vi "LVCAM Msg Drop.vi"(10 "Remaining Elements":refnum<class "Msg.lvclass">[](array[class]), 11 "Self Actor in":refnum<class "Self Actor.lvclass">) -> ()   [LabVIEW 2021, in "LVCAM.lvlib" / "Self Actor.lvclass"]
uses:
  Self Actor.lvclass
  Msg/Msg.lvclass
  Self Actor.lvclass/Self Actor.ctl
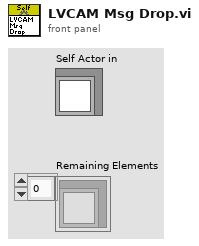
[diagram p1: front panel]
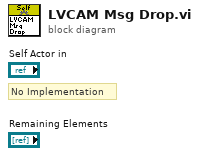
[diagram p0: block diagram]
diagram:
  # "No Implementation"
